vi "Simple_copy.vi"(6 "Angle 3":dbl(knob)=-72.06882847083946 scale=-90.0..90.0, 7 "L 3":dbl(slide)=10.0 scale=0.0..200.0, 8 "L 2":dbl(slide)=75.0 scale=0.0..200.0, 9 "L 1":dbl(slide)=75.0 scale=0.0..200.0, 10 "Angle 2":dbl(knob)=-72.06882847083946 scale=-90.0..90.0, 11 "Angle1":dbl(knob)=-45.83837436417874 scale=-90.0..90.0) -> (0 "Final 2D Pos":cluster{dbl, dbl}, 1 "end effector":cluster{dbl, dbl}={159.01647214211073, 1.9100783062530127} {"?" format="%.1f"; "?" format="%#.1f"}, 3 "2D Picture":picture)   [LabVIEW 2024]
panel:
  in  "2D Pict origin":cluster{"x":dbl, "y":dbl}={"x"=200.0, "y"=200.0}
  out "angle":dbl
  out "mag":dbl
  # "A 2"
  # "L1"
  # "L2"
  # "A 1"
  # "mm"
  # "mm"
  # "mm"
  # "mm"
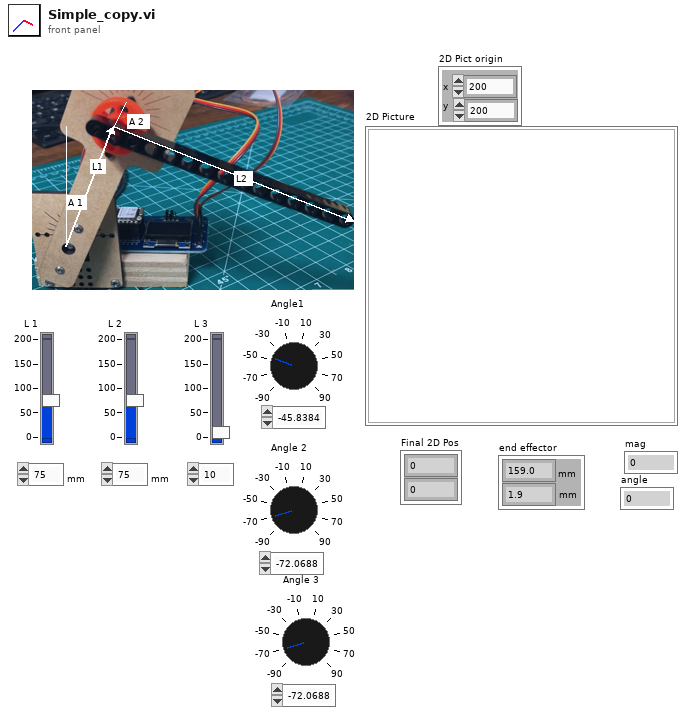
[diagram p1: front panel]
types:
  T1 = cluster{"Width":u16, "Style":enum32{"Solid", "Dash", "Dot", "DashDot", "DashDotDot"}}
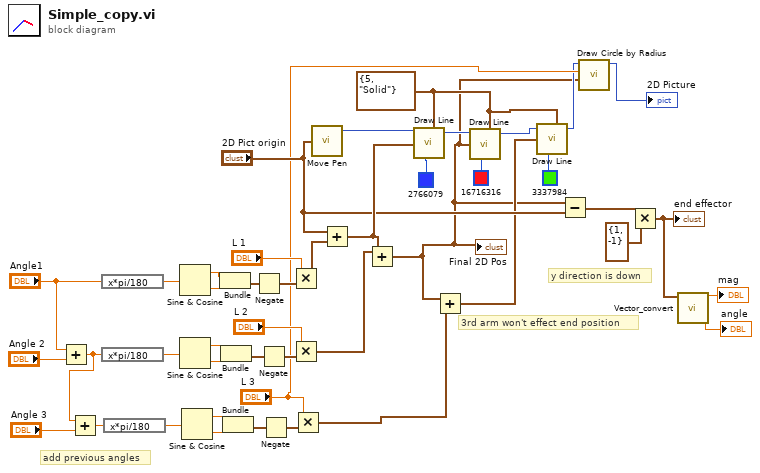
[diagram p0: block diagram]
diagram:
  w17 = T1 {"Width"=5, "Style"=enum."Solid"} ("pen")
  # "3rd arm won't effect end position"
  # "y direction is down"
  # "add previous angles"
  n1 = Add(x="Angle1", y="Angle 2") -> (x+y=w6:dbl)
  n2 = Add(x=w6, y="Angle 3") -> (x+y=w11:dbl)
  n3 = expression code="x*pi/180"("Angle1") -> (w43:dbl)
  n4 = expression code="x*pi/180"(w6) -> (w39:dbl)
  n5 = expression code="x*pi/180"(w11) -> (w13:dbl)
  n6 = Sine & Cosine(0:w43) -> (1:w27:dbl, 2:w26:dbl)
  n7 = Sine & Cosine(0:w39) -> (1:w24:dbl, 2:w23:dbl)
  n8 = Sine & Cosine(0:w13) -> (1:w10:dbl, 2:w9:dbl)
  n9 = Bundle(w27, w26) -> (w42:cluster{dbl, dbl})  [unwired: 1 in]
  n10 = Bundle(w24, w23) -> (w40:cluster{dbl, dbl})  [unwired: 1 in]
  n11 = Bundle(w10, w9) -> (w14:cluster{dbl, dbl})  [unwired: 1 in]
  n12 = Negate(x=w42) -> (-x=w25:cluster{dbl, dbl})
  n13 = Negate(x=w40) -> (-x=w22:cluster{dbl, dbl})
  n14 = Negate(x=w14) -> (-x=w8:cluster{dbl, dbl})
  n15 = Multiply(x="L 1", y=w25) -> (x*y=w41:cluster{dbl, dbl})
  n16 = Multiply(x="L 2", y=w22) -> (x*y=w37:cluster{dbl, dbl})
  n17 = Multiply(x="L 3", y=w8) -> (x*y=w7:cluster{dbl, dbl})
  n18 = call <vilib>:"Move Pen.vi"("new position"="2D Pict origin") -> ("new picture"=w44:picture)  [unwired: 4 in]
  n19 = Add(x="2D Pict origin", y=w41) -> (x+y=w36:cluster{dbl, dbl})
  n20 = Add(x=w37, y=w36) -> (x+y=w1:cluster{dbl, dbl})
  "Final 2D Pos" <- w1
  n21 = call <vilib>:"Draw Line.vi"("picture"=w44, "end point"=w36, "color(black)"=u32 2766079, "pen"=w17) -> ("new picture"=w38:picture)  [unwired: 5 in]
  n22 = Add(x=w1, y=w7) -> (x+y=w4:cluster{dbl, dbl})
  n23 = call <vilib>:"Draw Line.vi"("picture"=w38, "end point"=w1, "color(black)"=u32 16716316, "pen"=w17) -> ("new picture"=w15:picture)  [unwired: 5 in]
  n24 = call <vilib>:"Draw Line.vi"("picture"=w15, "end point"=w4, "color(black)"=u32 3337984, "pen"=w17) -> ("new picture"=w3:picture)  [unwired: 5 in]
  n25 = Subtract(x=w1, y="2D Pict origin") -> (x-y=w30:cluster{dbl, dbl})
  n26 = call <vilib>:"Draw Circle by Radius.vi"("pixel center"=w1, "radius"="L 3", "picture"=w3) -> ("new picture"=→"2D Picture":picture)  [unwired: 8 in]
  n27 = Multiply(x=w30, y=cluster{"x":i16, "y":i16} {"x"=1, "y"=-1} ("new position")) -> (x*y=w20:cluster{dbl, dbl})
  "end effector" <- w20
  n28 = call "Vector_convert.vi"("x,y"=w20) -> ("angle"=→"angle":dbl, "mag"=→"mag":dbl)  [unwired: 9 in]
